vi "App_SaveOnMP.vi"(11 "Spike":cluster{"Port":string, "All Code":string}) -> ()   [LabVIEW 2016]
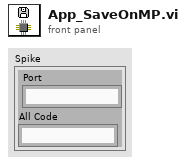
[diagram p1: front panel]
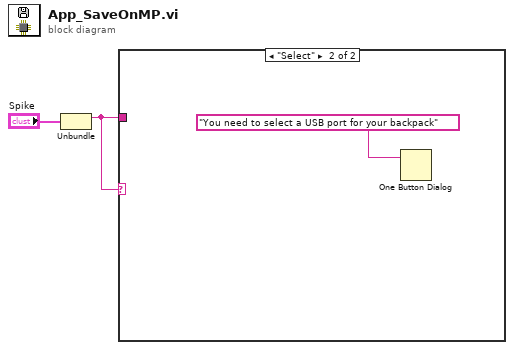
[diagram p0: block diagram]
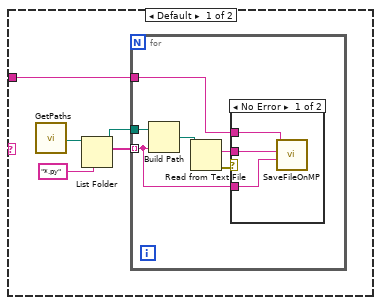
[diagram p2: hidden frame]
diagram:
  n1 = Unbundle("Spike") -> ("Port"=w1:string)  [unwired: 1 out]
  n2 = case shown="\"Select\"" w1 {
    tunnel: w1 -> [w3 _]
    frame Default {
      n3 = call "GetPaths.vi"() -> ("Libraries path"=w4:path)  [unwired: 10 in, 1 out]
      n4 = List Folder(path=w4, pattern="*.py") -> (path out=w7:path, filenames=w6:string[])  [unwired: 2 in, 2 out]
      n5 = for {
        tunnel: w6 -> [w10] mode=indexing
        tunnel: w7 -> [w13]
        tunnel: w3 -> [w8]
        n6 = Build Path(base path=w13, name or relative path=w10) -> (appended path=w12:path)
        n7 = Read from Text File(file (use dialog)=w12) -> (text=w11:string, error out=w9:errorcluster)  [unwired: 3 in, 2 out]
        n8 = case shown="No Error" w9 {
          tunnel: w8 -> [w16 _]
          tunnel: w11 -> [w15 _]
          tunnel: w10 -> [w14 _]
          frame No Error {
            n9 = call "SaveFileOnMP.vi"("FileName"=w14, "Code sent"=w15, "VISA in"=w16) -> ()  [unwired: 6 in, 3 out]
          }
          frame Error {
          }
        }
      }
    }
    frame "Select" {
      n10 = One Button Dialog(message="You need to select a USB port for your backpack") -> ()  [unwired: 1 in, 1 out]
    }
  }
